vi "Driver QL Series II.vi"() -> ()   [LabVIEW 2020]
panel:
  in  "Output on/off":bool
  in  "Output Channel":string
  out "error out":errorcluster
  in  "Current":string
  in  "Volts":string
  in  "VISA resource name":refnum<visa-resource-name>
  in  "error in (no error) 2":errorcluster
  in  "Voltage Channel":string
  in  "Current Channel":string
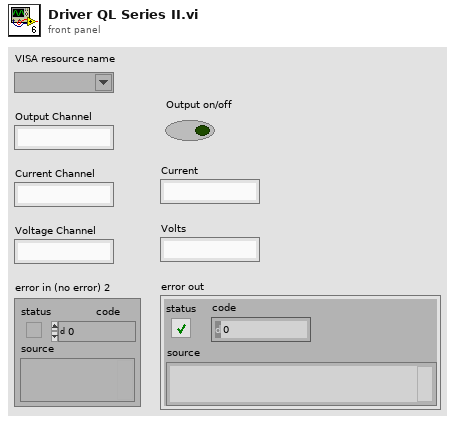
[diagram p1: front panel]
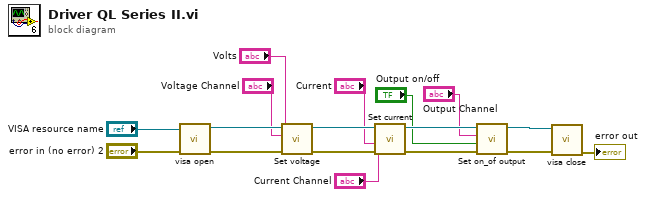
[diagram p0: block diagram]
diagram:
  n1 = call "visa open.vi"("error in (no error) 2"="error in (no error) 2", "VISA resource name"="VISA resource name") -> ("error out"=w12:errorcluster, "VISA resource name out"=w16:refnum<visa-resource-name>)  [unwired: 8 in]
  n2 = call "Set voltage.vi"("error in (no error)"=w12, "Volts"="Volts", "Channel"="Voltage Channel", "VISA resource name"=w16) -> ("error out"=w11:errorcluster, "VISA resource name out"=w15:refnum<visa-resource-name>)  [unwired: 6 in]
  n3 = call "Set current.vi"("error in (no error)"=w11, "Volts"="Current", "Channel"="Current Channel", "VISA resource name"=w15) -> ("error out"=w10:errorcluster, "VISA resource name out"=w14:refnum<visa-resource-name>)  [unwired: 6 in]
  n4 = call "Set on_of output.vi"("error in (no error)"=w10, "output on/off"="Output on/off", "Channel"="Output Channel", "VISA resource name"=w14) -> ("error out"=w9:errorcluster, "VISA resource name out"=w13:refnum<visa-resource-name>)  [unwired: 6 in]
  n5 = call "visa close.vi"("error in (no error)"=w9, "VISA resource name"=w13) -> ("error out"=→"error out":errorcluster)  [unwired: 9 in]
